vi "Init with Values.vi"(8 "error in":errorcluster, 10 "Values":variant, 11 "Combo Box in":refnum<class "Combo Box.lvclass">) -> (0 "error out":errorcluster, 3 "Combo Box out":refnum<class "Combo Box.lvclass">)   [LabVIEW 2024, in "SourceGrid.lvlib" / "Combo Box.lvclass"]
doc: "Values: ICollection compatible set of standard values"
uses:
  Combo Box.lvclass
  Combo Box.lvclass/Combo Box.ctl
  D:/git/Sourcegrid-LabVIEW/dll/SourceGrid.dll
  dll/SourceGrid.dll
  <vilib>/Utility/Data Type/NI_Data Type.lvlib
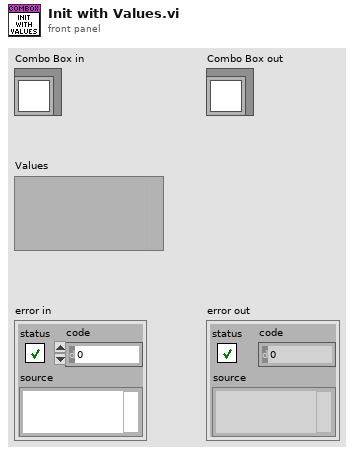
[diagram p1: front panel]
types:
  T1 = typedef "NI_Data Type.lvlib/Data Type.ctl" = enum8{"Invalid Type", "Void", "I8", "I16", "I32", "I64", "U8", "U16", "U32", "U64", "Single Float", "Double Float", "Extended Float", "Single Complex", "Double Complex", "Extended Complex", "Enum U8", "Enum U16", "Enum U32", "Enum U64", "Single Float With Unit", "Double Float With Unit", "Extended Float With Unit", "Single Complex with Unit", "Double Complex with Unit", "Extended Complex with Unit", "Boolean", "String", "Path", "Picture", "Tag", "Array", "Cluster", "Variant", "LV Variant", "Waveform", "Timestamp", "Digital Waveform", "Digital Data", "ExpressData", "Refnum", "External Data", "VI", "Poly VI", "LabVIEW Class Instance", "Fixed Point", "Set Collection", "Map Collection"}
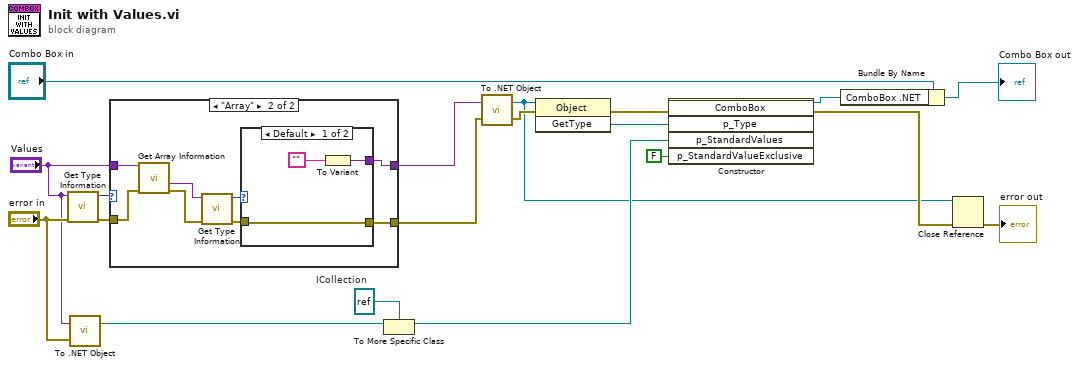
[diagram p0: block diagram]
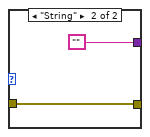
[diagram p3: hidden frame]
diagram:
  w9 = refnum<k24> refnum  # ICollection
  n1 = call <vilib>:"Get Type Information.vi"("error in (no error)"="error in", "variant"="Values") -> ("error out"=w18:errorcluster, "type"=w19:T1)  [unwired: 5 in, 3 out]
  n2 = call <vilib>:"To .NET Object.vi"("error in (no error)"="error in", "anything"="Values") -> (".NET object"=w13:refnum<k24>)  [unwired: 1 out]
  n3 = case shown="\"Array\"" w19 {
    tunnel: w18 -> [w21 w27]
    tunnel: "Values" -> [w20 w29]
    tunnel: [w20 w23] -> w16
    tunnel: [w21 w22] -> w15
    frame Default {
    }
    frame "Array" {
      n4 = call <vilib>:"Get Array Information.vi"("error in (no error)"=w27, "variant"=w29) -> ("error out"=w26:errorcluster, "array element data type"=w24:variant)  [unwired: 6 in, 2 out]
      n5 = call <vilib>:"Get Type Information.vi"("error in (no error)"=w26, "variant"=w24) -> ("error out"=w25:errorcluster, "type"=w28:T1)  [unwired: 5 in, 3 out]
      n6 = case shown="Default" w28 {
        tunnel: w25 -> [w32 w34]
        tunnel: [w32 w34] -> w22
        tunnel: [w30 ""] -> w23
        frame Default {
          n7 = To Variant(anything="") -> (Variant=w30:variant)
        }
        frame "String" {
        }
      }
    }
  }
  n8 = To More Specific Class(target class=w9, reference=w13) -> (specific class reference=w10:refnum<k24>)  [unwired: 1 in, 1 out]
  n9 = call <vilib>:"To .NET Object.vi"("error in (no error)"=w15, "anything"=w16) -> ("error out"=w14:errorcluster, ".NET object"=w1:refnum<k24>)
  n10 = invoke class="Object" method="GetType"(reference=w1, error in=w14) -> (error out=w7:errorcluster, "GetType"=w17:refnum<k24>)  [unwired: 1 in, 1 out]
  n11 = constructor class="ComboBox"(error in=w7, "p_Type"=w17, "p_StandardValues"=w10, "p_StandardValueExclusive"=FALSE) -> (reference out=w4:refnum<k24>, error out=w6:errorcluster)  [unwired: 2 in, 4 out]
  n12 = Bundle By Name(cluster="Combo Box in", "ComboBox .NET"=w4) -> (→"Combo Box out":refnum<class "Combo Box.lvclass">)
  n13 = Close Reference(reference=w1, error in (no error)=w6) -> (error out=→"error out":errorcluster)
